vi "Register Configuration and Results.vi"(8 "error in (no error)":errorcluster, 10 "Measurement":refnum<class "MeasurementPluginService.lvclass">, 11 "gRPC ID":T1) -> (0 "error out":errorcluster, 3 "gRPC ID Out":T1)   [LabVIEW 2020, in "MeasurementLink Measurement Server.lvlib"]
uses:
  MeasurementLink Measurement Server.lvlib
  <vilib>/gRPC/LabVIEW gRPC Library/Shared/grpcId.ctl
  RPC Service/MeasurementService/MeasurementPluginService.lvclass
  <vilib>/gRPC/LabVIEW gRPC Library/grpc-lvsupport-release.lvlib
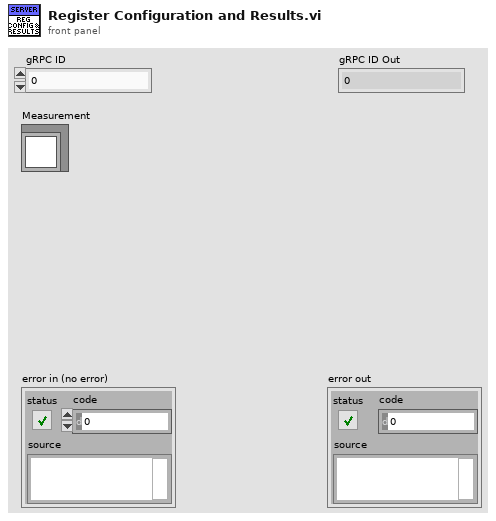
[diagram p1: front panel]
types:
  T1 = typedef "grpc-lvsupport-release.lvlib/grpcId.ctl" = u64
  T2 = typedef "grpc-lvsupport-release.lvlib/Message Metadata.ctl" = cluster{"Version":i32, "Name":string, "Type Url":string, "Elements":T3[]}
  T3 = typedef "grpc-lvsupport-release.lvlib/Message Element Metadata.ctl" = cluster{"Embedded Message Name":string, "Protobuf Index":i32, "MessageElementType":T4, "Repeated":bool}
  T4 = typedef "grpc-lvsupport-release.lvlib/Message Element Type.ctl" = enum32{"Int32Value", "FloatValue", "DoubleValue", "BoolValue", "StringValue", "MessageValue", "Int64Value", "UInt32Value", "UInt64Value", "EnumValue", "Bytes", "Fixed64", "Fixed32", "SFixed64", "SFixed32", "SInt64", "SInt32"}
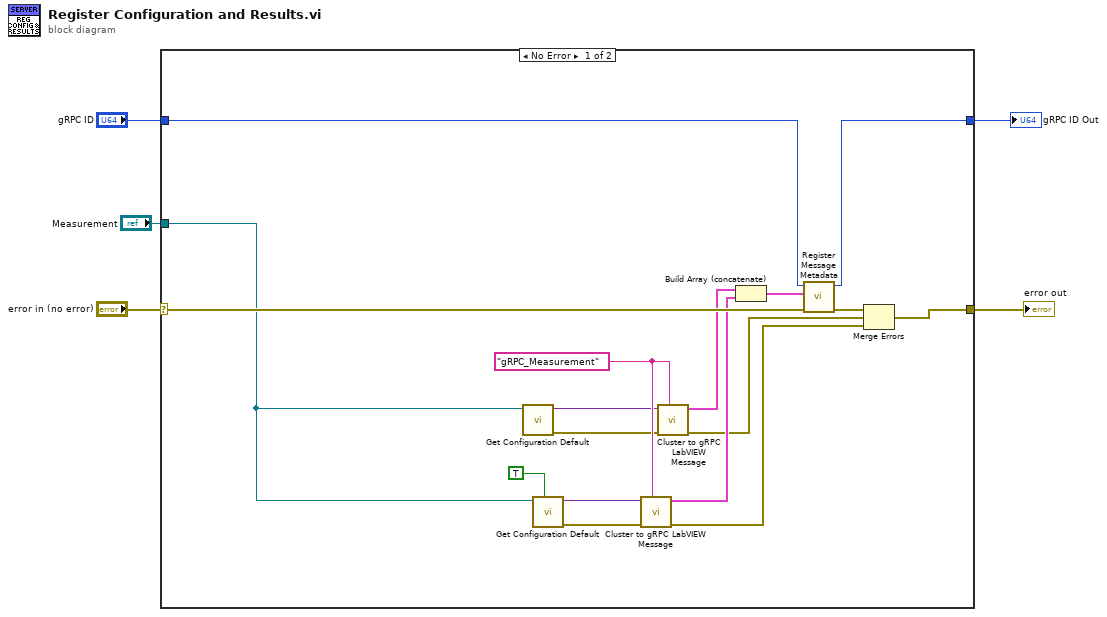
[diagram p0: block diagram]
diagram:
  n1 = case shown="No Error" "error in (no error)" {
    selector: "error in (no error)" -> [w21 w24]
    tunnel: [w14 w23] -> w2
    tunnel: [w17 w24] -> w5
    tunnel: "gRPC ID" -> [w13 w23]
    tunnel: "Measurement" -> [w6 _]
    frame No Error {
      w12 = "gRPC_Measurement" ("Package Name")
      n2 = call "Get Configuration Default.vi"("Measurement"=w6) -> ("error out"=w10:errorcluster, "Control Default"=w11:variant)  [unwired: 9 in]
      n3 = call "Get Configuration Default.vi"("Get Results Default? (F)"=TRUE, "Measurement"=w6) -> ("error out"=w7:errorcluster, "Control Default"=w9:variant)  [unwired: 8 in]
      n4 = call <vilib>:"Cluster to gRPC LabVIEW Message.vi"("Package Name"=w12, "error in"=w7, "Cluster"=w9) -> ("error out"=w16:errorcluster, "gRPC Message Metadata []"=w19:T2[])  [unwired: 7 in]
      n5 = call <vilib>:"Cluster to gRPC LabVIEW Message.vi"("Package Name"=w12, "error in"=w10, "Cluster"=w11) -> ("error out"=w15:errorcluster, "gRPC Message Metadata []"=w20:T2[])  [unwired: 7 in]
      n6 = Build Array (concatenate)(w20, w19) -> (w18:T2[])
      n7 = call <vilib>:"Register Message Metadata.vi"("error in"=w21, "Messages"=w18, "gRPCid in"=w13) -> ("error out"=w22:errorcluster, "gRPCid out"=w14:T1)  [unwired: 7 in]
      n8 = Merge Errors(w22, w15, w16) -> (w17:errorcluster)
    }
    frame Error {
    }
  }
  "error out" <- w5
  "gRPC ID Out" <- w2
